vi "Test Error Handler Interface Handle Errors.vi"(8 "error in (no error)":errorcluster, 11 "Test Case In":refnum<class "Error Handler Interface Test.lvclass">) -> (0 "error out":errorcluster, 3 "Test Case Out":refnum<class "Error Handler Interface Test.lvclass">)   [LabVIEW 2020, in "Error Handler Interface Test.lvclass"]
uses:
  Error Handler Interface Test.lvclass
  C:/Program Files (x86)/National Instruments/LabVIEW 2020/vi.lib/Astemes/LUnit/Test Case.lvclass
  Error Handler Interface Test.lvclass/Error Handler Interface Test.ctl
  <vilib>/Astemes/LUnit/Test Case.lvclass/Test Case.ctl
  <vilib>/Astemes/LUnit/LUnit Assertion Result.lvclass/LUnit Assertion Result.ctl
  <vilib>/Astemes/LUnit/LUnit Test Case Result.lvclass/LUnit Test Case Result.ctl
  <vilib>/Astemes/LUnit/LUnit Method Result.lvclass/LUnit Method Result.ctl
  <vilib>/Astemes/LUnit/Palette/Pass.vi
  <vilib>/Astemes/LUnit/Palette/Fail.vi
  <vilib>/Astemes/LUnit/Set Assertion Type.vi
  <vilib>/Astemes/LUnit/Add test result.vi
  <vilib>/Astemes/LUnit/LUnit Write Passed.vi
  <vilib>/Astemes/LUnit/LUnit Write Message.vi
  <vilib>/Astemes/LUnit/LUnit Write Description.vi
  <vilib>/Astemes/LUnit/LUnit Write Assertion Type.vi
  <vilib>/Astemes/LUnit/LUnit Record Assertion Result.vi
  <vilib>/Astemes/LUnit/LUnit Aggregate Assertion Results.vi
  <vilib>/Astemes/LUnit/Assertion Result/LUnit Read Status.vi
  <vilib>/Astemes/LUnit/LUnit Read Message.vi
  <vilib>/Astemes/LUnit/LUnit Read Description.vi
  <vilib>/Astemes/LUnit/Method Result/LUnit Merge Status.vi
  <vilib>/Astemes/LUnit/LUnit Concatenate result strings.vi
  Framework/Error Handler Interface/Error Handler Interface.lvclass
  <vilib>/Astemes/LUnit/LUnit Assertion Result.lvclass
  <vilib>/Astemes/LUnit/Test Case.lvclass
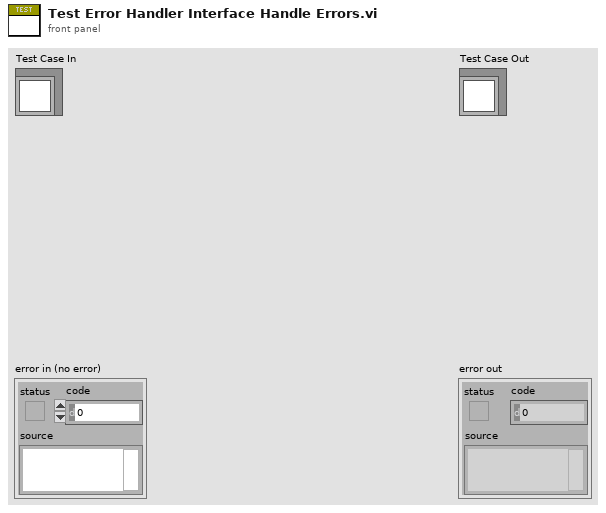
[diagram p1: front panel]
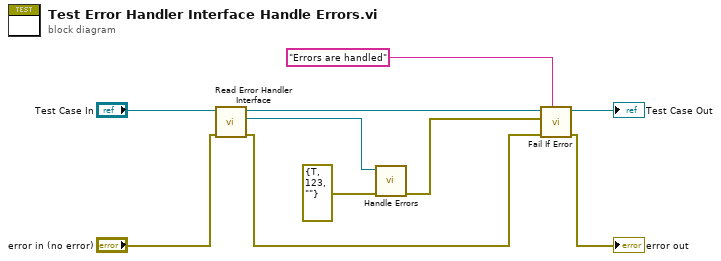
[diagram p0: block diagram]
diagram:
  n1 = call "Read Error Handler Interface.vi"("error in (no error)"="error in (no error)", "Error Handler Interface Test in"="Test Case In") -> ("error out"=w2:errorcluster, "Error Handler Interface"=w7:refnum<class "Error Handler Interface.lvclass">, "Error Handler Interface Test out"=w8:refnum<class "Error Handler Interface Test.lvclass">)  [unwired: 7 in]
  n2 = call-dynamic "Handle Errors.vi"("error in (no error)"=errorcluster {"status"=TRUE, "code"=123, "source"=""}, "Error Handler Interface In"=w7) -> ("error out"=w4:errorcluster)  [unwired: 8 in, 1 out]
  n3 = call <vilib>:"Fail If Error.vi"("Description"="Errors are handled", "error in (no error)"=w2, "Assert error"=w4, "LUnit Test Case In"=w8) -> ("error out"=→"error out":errorcluster, "LUnit Test Case Out"=→"Test Case Out":refnum<class "Error Handler Interface Test.lvclass">)  [unwired: 6 in]
